vi "FGV-MassData(lvlibp).vi"(6 "Operation":T1, 8 "Error in":errorcluster caption="Error in (no error)", 9 "size":i32, 10 "Start":i32, 11 "Data in":u8[](array[numeric])) -> (0 "Error out":errorcluster, 1 "Active Read Oper":T2, 2 "Active Write Oper":T2, 3 "Data out":u8[](array[numeric]))   [LabVIEW 2017, in "CSM MassData Parameter Support.lvlib"]
uses:
  CSM MassData Parameter Support.lvlib
  Def-MassDataOper-Status.ctl
  Operation-FGV-MassData.ctl
  FGV-MassData.vi
  <userlib>/_NEVSTOP/Communicable State Machine(CSM)/Communicable State Machine.lvlib
  <userlib>/_NEVSTOP/Communicable State Machine(CSM)/_Shared/CSM Shared.lvlib
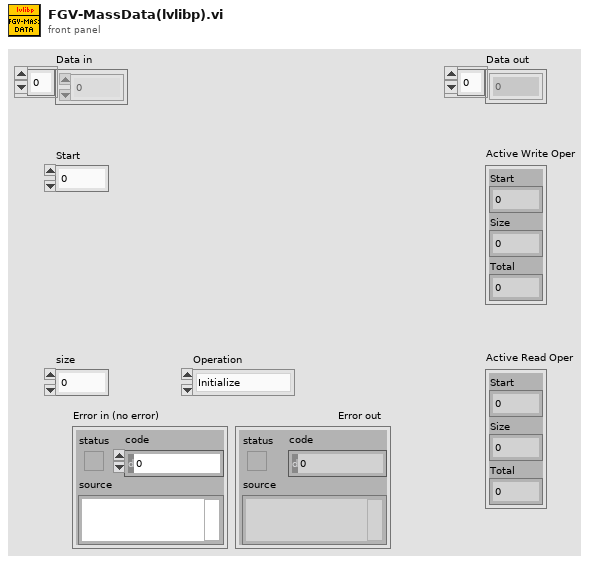
[diagram p1: front panel]
types:
  T1 = typedef "CSM MassData Parameter Support.lvlib/Operation-FGV-MassData.ctl" = enum16{"Initialize", "Read", "Write", "Status", "Release"}
  T2 = typedef "CSM MassData Parameter Support.lvlib/Def-MassDataOper-Status.ctl" = cluster{"Start":i32, "Size":i32, "Total":i32}
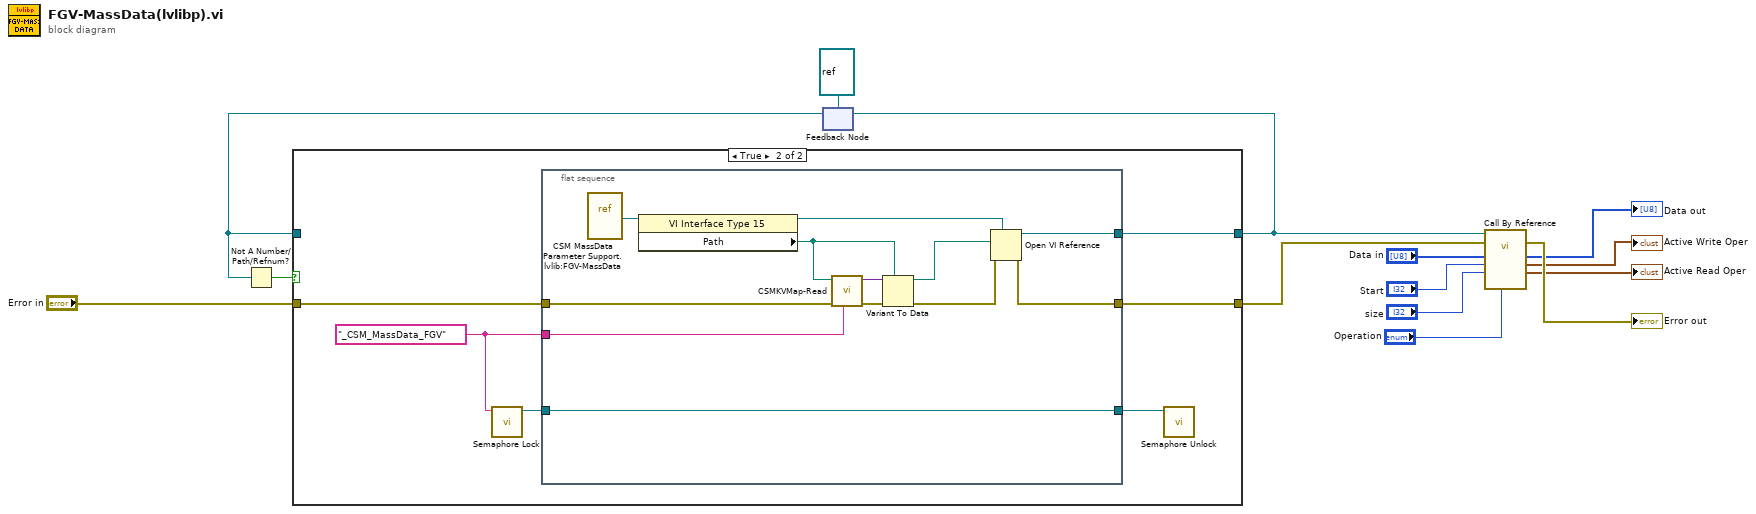
[diagram p0: block diagram]
diagram:
  n1 = feedback #1(refnum<vi> refnum) -> (w12:refnum<vi>)
  n2 = Not A Number/Path/Refnum?(number/path/refnum=w12) -> (NaN/Path/Refnum?=w13:bool)
  n3 = case shown="True" w13 {
    tunnel: [w16 w22] -> w11
    tunnel: w12 -> [w16 _]
    tunnel: "Error in" -> [w15 w21]
    tunnel: [w15 w20] -> w9
    frame False {
    }
    frame True {
      w17 = "_CSM_MassData_FGV" ("name")
      n4 = call <userlib>:"Semaphore Lock.vi"("name"=w17) -> ("semaphore"=w18:refnum<queue>)  [unwired: 10 in]
      n5 = flat-sequence {
        tunnel: [w27] -> w22
        tunnel: w21 -> [w26]
        tunnel: [w23] -> w20
        tunnel: w17 -> [w24]
        tunnel: [w25] -> w19
        tunnel: w18 -> [w25]
        frame #0 {
          n6 = vi-ref "CSM MassData Parameter Support.lvlib:FGV-MassData.vi"() -> (w34:refnum<vi>)
          n7 = property class="VI Interface Type 15"(reference=w34) -> (reference out=w28:refnum<vi>, "Path"=w31:path)  [unwired: 1 in, 1 out]
          n8 = call <userlib>:"CSMKVMap-Read.vi"("name"=w24, "Error in"=w26, "default value (empty variant)"=w31) -> ("Error out"=w33:errorcluster, "value"=w32:variant)  [unwired: 5 in]
          n9 = Variant To Data(error in=w33, type=w31, Variant=w32) -> (data=w30:path, error out=w29:errorcluster)
          n10 = Open VI Reference(type specifier VI Refnum (for type only)=w28, vi path=w30, error in (no error)=w29) -> (vi reference=w27:refnum<vi>, error out=w23:errorcluster)  [unwired: 3 in]
        }
      }
      n11 = call <userlib>:"Semaphore Unlock.vi"("semaphore"=w19) -> ()  [unwired: 11 in]
    }
  }
  n12 = feedback-in #1(w11) -> ()
  n13 = call-by-ref "?"(reference=w11, error in=w9, "Operation"="Operation", "size"="size", "Start"="Start", "Data in"="Data in") -> (error out=→"Error out":errorcluster, "Active Read Oper"=→"Active Read Oper":T2, "Active Write Oper"=→"Active Write Oper":T2, "Data out"=→"Data out":u8[])  [unwired: 4 in, 2 out]
